vi "Global Variables.vi"() -> ()   [LabVIEW 2018]
uses:
  Controls/Optimization Type Selector.ctl
panel:
  in  "Enable Remote Operation":bool
  in  "Networked?":bool
  in  "Optimization Type":T1
  in  "Per-Unitize?":bool
  in  "Dev Env?":bool=TRUE
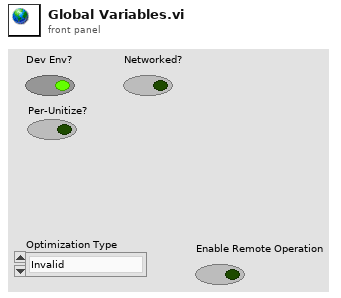
[diagram p1: front panel]
types:
  T1 = typedef "Optimization Type Selector.ctl" = enum16{"Invalid", "Single Phase", "Volttron"}
diagram:
